vi "(範例)2D Serial Robot Animation.vi"() -> ()   [LabVIEW 2015]
doc: "This VI animates a robotic arm using a 2D Picture. By changing the knobs and sliders, you can change the lengths and angles of the various components of the arm."
panel:
  in  "Base position Y":dbl(slide)=100.0
  in  "Base position X":dbl(slide)=50.0 scale=0.0..100.0
  in  "Scale Factor":dbl(slide)=0.7 scale=0.5..1.0
  in  "Light Direction":dbl(knob)=5.611498737356196 scale format="%#.1f"
  in  "Add details":bool=TRUE
  in  "Joint C":dbl(knob)=5.611498737356196 scale format="%#.1f"
  in  "Claw Value":dbl(slide)=1.0 scale=0.0..1.0
  in  "Colors":T1={"Joint A"=16750848, "Arm A"=16764006, "Joint B"=26316, "Arm B"=6723993, "Joint C"=16724787, "Claw"=16776960}
  in  "Joint B":dbl(knob)=5.611498737356196 scale format="%#.1f"
  in  "Joint A":dbl(knob)=5.611498737356196 scale format="%#.1f"
  in  "Length B":dbl(slide)=35.714285714285715 scale=10.0..80.0
  in  "Length A":dbl(slide)=70.71428571428572 scale=10.0..80.0
  in  "Stop":bool
  out "Picture":picture
  # "Overview: This VI demonstrates how to animate a robotic arm using a 2D Picture.\nInstructions: \n1. Run the VI.\n2. Change the Base position X and Base position Y sliders to define the position of the arm.\n3. Change the Length A and Length B sliders to define the size of the arm.\n4. Change the Joint A, Joint B, and Joint C knobs to rotate the arm.\n5. Change the Claw Value slider to open and close the claw.\n6. Click Stop to stop the VI."
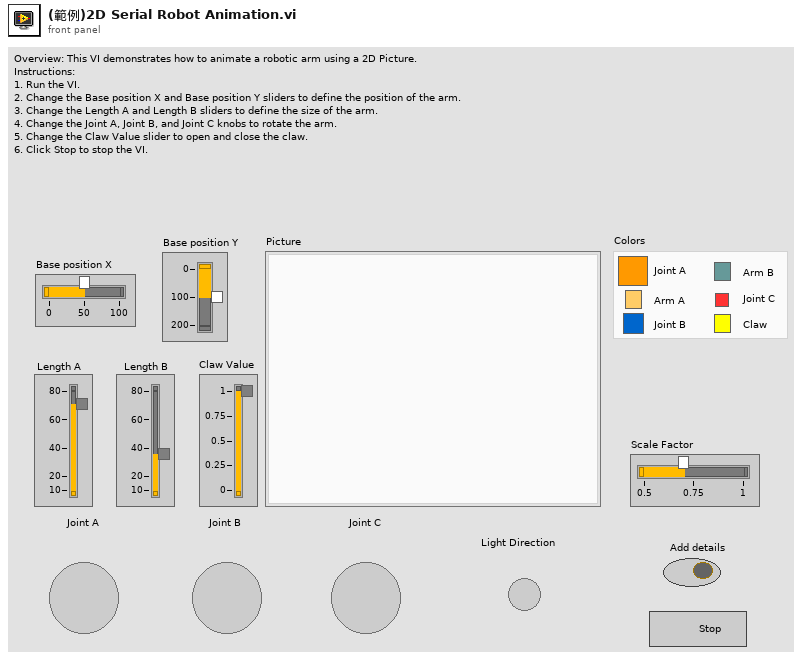
[diagram p1: front panel]
types:
  T1 = cluster{"Joint A":u32, "Arm A":u32, "Joint B":u32, "Arm B":u32, "Joint C":u32, "Claw":u32}
  T2 = cluster{"top":dbl, "left":dbl, "height":dbl, "width":dbl}
  T3 = cluster{"Joint A":dbl, "height":dbl, "Scale Factor":dbl}
  T4 = cluster{"left":dbl, "top":dbl, "right":dbl, "bottom":dbl}
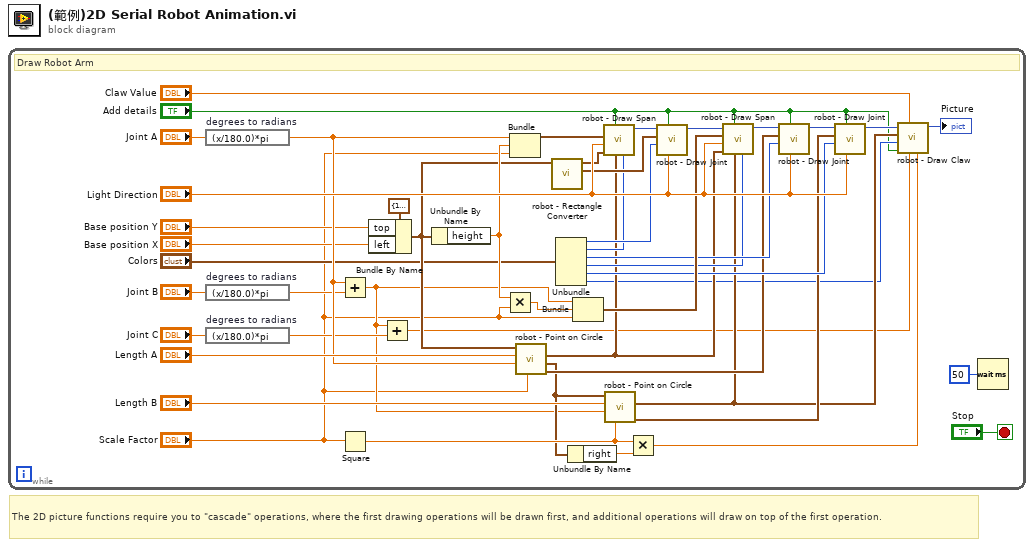
[diagram p0: block diagram]
diagram:
  # "The 2D picture functions require you to \"cascade\" operations, where the first drawing operations will be drawn first, and additional operations will draw on top of the first operation."
  n1 = while {
    stop <- "Stop" stop-if-true
    # "Draw Robot Arm"
    n2 = expression code="(x/180.0)*pi" "degrees to radians"("Joint A") -> (w26:dbl)
    n3 = expression code="(x/180.0)*pi" "degrees to radians"("Joint B") -> (w21:dbl)
    n4 = expression code="(x/180.0)*pi" "degrees to radians"("Joint C") -> (w25:dbl)
    n5 = Add(x=w26, y=w21) -> (x+y=w2:dbl)
    n6 = Square(x="Scale Factor") -> (x^2=w18:dbl)
    n7 = Bundle By Name(cluster=T2 {"top"=120.0, "left"=70.0, "height"=32.0, "width"=32.0} ("Circle"), "top"="Base position Y", "left"="Base position X") -> (w20:T2)
    n8 = Add(x=w2, y=w25) -> (x+y=w11:dbl)
    n9 = Unbundle By Name(w20) -> ("height"=w41:dbl)
    n10 = Multiply(x=w41, y="Scale Factor") -> (x*y=w44:dbl)
    n11 = Bundle("Joint A"=w26, "height"=w41, "Scale Factor"="Scale Factor") -> (w42:T3)  [unwired: 1 in]
    n12 = call "robot - Point on Circle.vi"("Scale Factor"="Scale Factor", "Angle"=w26, "Radius"="Length A", "Rect In"=w20) -> ("Scaled Rect Out"=w15:T4, "Rect Out"=w14:T4, "scaled point"=w16:cluster{"x":dbl, "y":dbl})  [unwired: 4 in, 1 out]
    n13 = call "robot - Rectangle Converter.vi"("Rect"=w20) -> ("Rect Out"=w35:T4, "Center"=w19:cluster{"x":dbl, "y":dbl})  [unwired: 9 in]
    n14 = Unbundle("Colors") -> ("Joint A"=w36:u32, "Arm A"=w33:u32, "Joint B"=w37:u32, "Arm B"=w32:u32, "Joint C"=w38:u32, "Claw"=w6:u32)
    n15 = Unbundle By Name(w14) -> ("right"=w34:dbl)
    n16 = Bundle(w2, w44, "Scale Factor"="Scale Factor") -> (w43:cluster{dbl, dbl, "Scale Factor":dbl})  [unwired: 1 in]
    n17 = call "robot - Draw Span.vi"("Color"=w33, "Center 2"=w16, "Enhance Style"="Add details", "Center 1"=w19, "Light Direction"="Light Direction", "Circle Spec"=w42) -> ("Picture Out"=w39:picture)  [unwired: 5 in]
    n18 = call "robot - Point on Circle.vi"("Scale Factor"=w18, "Angle"=w2, "Radius"="Length B", "Rect In"=w14) -> ("Scaled Rect Out"=w17:T4, "scaled point"=w13:cluster{"x":dbl, "y":dbl})  [unwired: 4 in, 2 out]
    n19 = Multiply(x=w18, y=w34) -> (x*y=w7:dbl)
    n20 = call "robot - Draw Joint.vi"("Light Direction"="Light Direction", "Enhance Style"="Add details", "Color"=w36, "Rectangle"=w35, "Picture In"=w39) -> ("Picture Out"=w10:picture)  [unwired: 6 in]
    n21 = call "robot - Draw Span.vi"("Color"=w32, "Center 2"=w13, "Enhance Style"="Add details", "Center 1"=w16, "Light Direction"="Light Direction", "Circle Spec"=w43, "Picture In"=w10) -> ("Picture Out"=w40:picture)  [unwired: 4 in]
    n22 = call "robot - Draw Joint.vi"("Light Direction"="Light Direction", "Enhance Style"="Add details", "Color"=w37, "Rectangle"=w15, "Picture In"=w40) -> ("Picture Out"=w9:picture)  [unwired: 6 in]
    n23 = call "robot - Draw Joint.vi"("Light Direction"="Light Direction", "Enhance Style"="Add details", "Color"=w38, "Rectangle"=w17, "Picture In"=w9) -> ("Picture Out"=w8:picture)  [unwired: 6 in]
    n24 = call "robot - Draw Claw.vi"("Diameter"=w7, "Claw Angle"=w11, "Claw Value"="Claw Value", "Enhance Style"="Add details", "Claw Color"=w6, "Position"=w13, "Picture In"=w8) -> ("Picture Out"=→"Picture":picture)  [unwired: 4 in]
    n25 = Wait (ms)(milliseconds to wait=u32 50) -> ()  [unwired: 1 out]
  }
